vi "AlliGator Select Source Image ROI.vi"(8 "Error In":errorcluster, 11 "ROI Selection Data":T1) -> (0 "Error Out":errorcluster, 1 "Overlay Color":u32(colorbox), 2 "ROI Name":string, 3 "ROI Descriptor":T3 {"Contours"."Type" items=["No Selection", "Point", "Line", "Rectangle", "Oval", "Polygon", "Freehand Region", "Annulus", "Unused2", "Unused3", "Broken Line", "Freehand Line", "Rotated Rectangle"]}, 4 "Current ROI":i32, 5 "# ROIs":i32)   [LabVIEW 2021, in "AlliGator ROIs.lvlib"]
doc: "Selects Source Image ROI(s)."
uses:
  AlliGator ROIs.lvlib
  AlliGator ROI Selection Data.ctl
  AlliGator ROI Manager Actions.ctl
  Globals, Variables, Constants/AlliGator Variables List.ctl
  Image/Named ROI Description.ctl
  Variant/Variant to Data/Variant to I32.vi
  <userlib>/_OpenG.lib/string/string.llb/openg_string.lvlib
  Globals, Variables, Constants/AlliGator Globals, Variables & Constants.lvlib
  Image/Image.lvlib
  Variant/Variant to Data/Variant to Data.lvlib
  Arrays/Arrays.lvlib
  Utilities/Utilities.lvlib
  Time/Time.lvlib
panel:
  # "see the AlliGator License on the block diagram (Ctrl+E or Window:Show Block Diagram)"
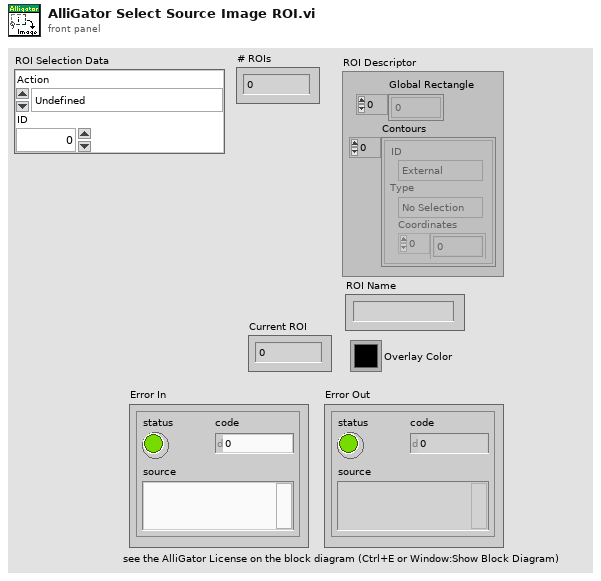
[diagram p1: front panel]
types:
  T1 = typedef "AlliGator ROIs.lvlib/AlliGator ROI Selection Data.ctl" = cluster{"Action":T2, "ID":i32}
  T2 = typedef "AlliGator ROIs.lvlib/AlliGator ROI Manager Actions.ctl" = enum16{"Undefined", "Delete Current ROI", "Delete All Unselected ROIs", "Delete Multiple ROIs", "Delete All ROIs", "Swap ROIs", "Insert ROI", "Update Current ROI Descriptor", "Rename Current ROI", "Store New ROI", "Store Multiple ROIs", "Select Next ROI", "Select Previous ROI", "Find Selected ROI", "Show All ROIs", "Update ROI Manager Window", "Merge All ROIs", "Unmerge ROI", "Set Selected ROI by ID"}
  T3 = typedef "ROI Descriptor" = cluster{"Global Rectangle":i32[], "Contours":cluster{"ID":enum32{"External", "Internal"}, "Type":u32, "Coordinates":i32[]}[]}
  T4 = typedef "AlliGator Globals, Variables & Constants.lvlib/AlliGator Variables List.ctl" = enum16{"---- GUI ----", "GUI:Initialization Status", "GUI:State Indicators Refnum", "GUI:Original AlliGator Menu Items", "GUI:Current Action Loop State", "GUI:Script in progress", "GUI:Playback", "GUI:Loop Playback", "GUI:Search ROI Used", "GUI:Search ROI", "Decay Graph Max Legend Size", "Intensity Graph Max Legend Size", "Decay Statistics Graph Max Legend Size", "Phasor Graph Max Legend Size", "Phasor Ratio Graph Max Legend Size", "Lifetime Graph Max Legend Size", "---- Files ----", "Files:Export Dataset Frames as Individual Files", "Files:Show Batch Export Help Balloons", "Files:Frames in Dataset", "Files:ptu File Frame Start Indices", "Files:Current Frame in Dataset", "Files:Current Frame Timestamp", "Files:Dataset Loaded", "Files:Dataset Metadata", "Files:Dataset Channel", "Files:Dataset Data Description", "Files:Background Dataset Metadata", "Files:Background Dataset Channel", "Files:Background Dataset Data Description", "Files:Background File Subtraction", "Files:Background File Path", "Files:Background File Pile-up Correction", "Files:Background File Pixel Well Capacity", "Files:Background File Scaling Factor", "Files:Current Dataset Load Settings", "Files:Dataset Path", "Files:ICCD-specific Information", "Files:Macrotime Gate Separation", "------ Python Plugins ------", "Python Plugins:Information", "Python Plugins:Python Session", "Python Plugins:Valid Python Session?", "---- Source Image ----", "Source Image:ROIs", "Source Image:Current ROI", "Source Image:ROI Event Refnum", "X_Source Image Display Range", "X_Source Image Palette Information", "X_Type of Displayed Image", "X_Time Gate Slider", "Source Image:Palette List", "Source Image:Scale", "Source Image:ROI Overlay Color", "Source Image:Overlay to Erase", "Source Image:Is Displayed Image Accumulated", "Source Image:White Light Image Modified", "Source Image:Mask Image Modified", "---- Image Profile Window ----", "Image Profile:Window Event Refnum", "Image Profile:IntensityType", "Image Profile:Intensity Average Type", "Image Profile:Intensity-weighted SDV", "Image Profile:Box Profile Type", "Image Profile:Window Open", "Image Profile:Plotted Fit Parameter", "------ Phasor Graph -------", "Phasor Graph:Show Line", "---- Phasor Plot ---", "Phasor Plot:Parameters Changed", "Phasor Plot:FLI Dataset Modified since last Calculation", "Phasor Harmonics Data", "Selected Phasor Harmonics", "Phasor Harmonic Manager Event Refnum", "Phasor Plot:ROIs", "Phasor Plot:Current ROI", "Phasor Plot:ROI Event Refnum", "Phasor Plot:Image Reference Points", "Phasor Plot:Computed", "Phasor Plot:Palette Information", "Phasor Plot:Palette List", "Phasor Plot:Phasor Ratio Palette Information", "Phasor Plot:Phasor Ratio Palette List", "Phasor Plot:Image Scale", "Phasor Plot:Image Overlay to Erase", "Phasor Plot:Image Elements to Update", "Phasor Plot:Current Calculation Parameters", "Phasor Plot:Current Calibration Options", "Phasor Plot:Reset Cumulated Phasor Plot", "Phasor Plot:Reference 1", "Phasor Plot:Lifetime Reference 1", "Phasor Plot:Reference 1 Frequency", "Phasor Plot:Reference 2", "Phasor Plot:Lifetime Reference 2", "Phasor Plot:Reference 2 Frequency", "---- Decay Analysis ----", "Number of Selected Decays to Fit", "LS Fit Results", "LAR Fit Results", "BS Fit Results", "Last Decay Max - Min", "Best Fit Parameters", "Best Fit Parameter Names", "Actual Size X", "Actual Size Y", "Binning X", "Binning Y", "Actual # Gates", "Dataset Number", "Gates to...", "Gates Skipped", "Gates to keep", "Gate Step", "Gate Separation", "Reversed Gates", "Pile-up Correction", "Pixel Well Capacity", "Background Subtracted", "Background Subtraction Method", "Background Definition Range", "Background File (deprecated)", "Number of Dataset Accumulated", "Array of Accumulated Dataset Paths", "Do Averaged Datasets", "Destination File Path", "Process Plot Target", "Use 1/D as Phasor Frequency", "---- Decay Fit Parameter Map -----", "Decay Fit Parameter Map:Palette Information", "Decay Fit Parameter Map:Palette List", "---- Parameter Map ----", "Parameter Map:Palette Information", "Parameter Map:Palette List", "------- Local Decay Window ---------", "Local Decay Graph Window:Event Refnum", "Local Decay Graph Window:Use normalized IRF for convolution", "----- Miscellaneous ----", "Misc:Skippable Dialog Windows Status"}
  T5 = typedef "Image.lvlib/Named ROI Description.ctl" = cluster{"ROI Descriptor":T3, "ROI Name":string, "Overlay Color":u32}
  T6 = typedef "AlliGator ROIs.lvlib/AlliGator Image ROI Event refnum.ctl" = refnum<user-event>
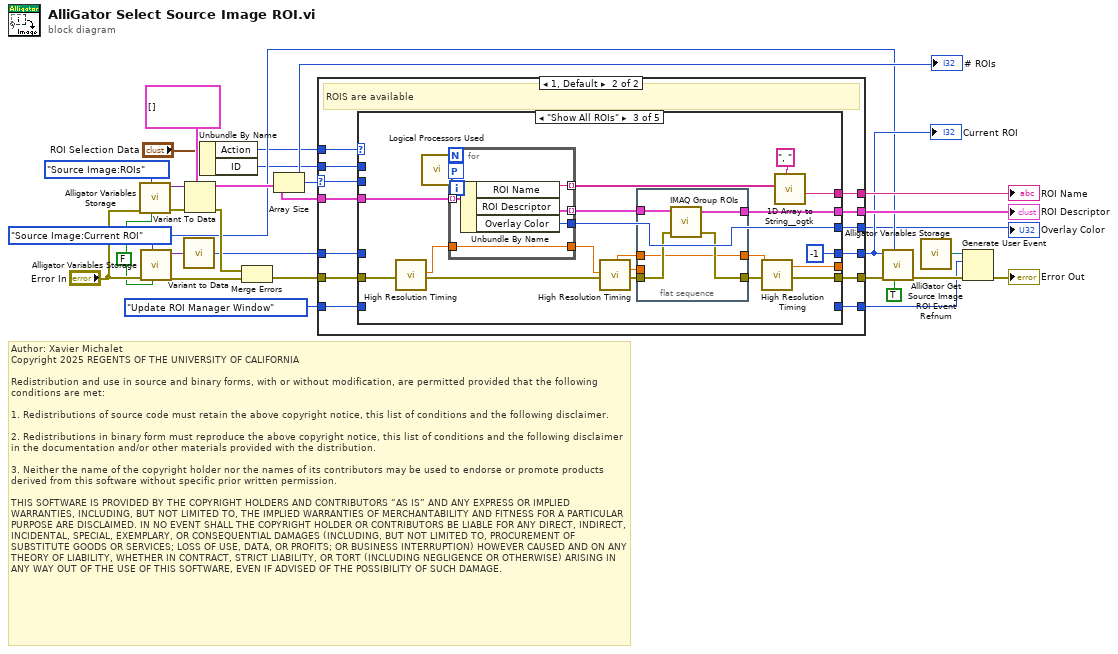
[diagram p0: block diagram]
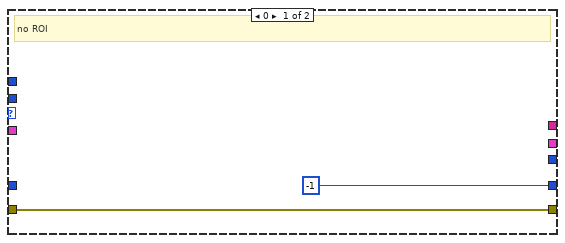
[diagram p2: hidden frame]
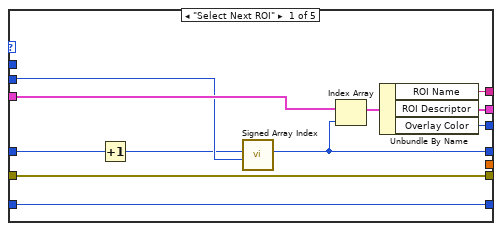
[diagram p3: hidden frame]
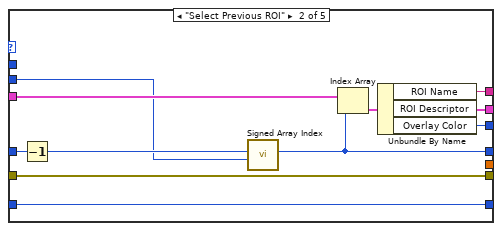
[diagram p4: hidden frame]
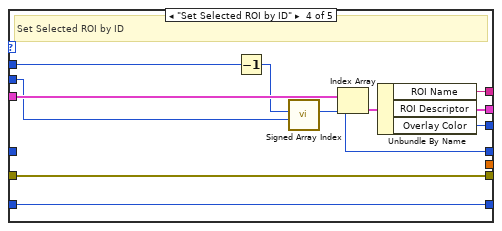
[diagram p5: hidden frame]
diagram:
  w11 = AlliGator_Variables_List."Source Image:Current ROI" ("Alligator Variable")
  w18 = FALSE ("Get(F)/Set")
  # "Author: Xavier Michalet\nCopyright 2025 REGENTS OF THE UNIVERSITY OF CALIFORNIA\n\nRedistribution and use in source and binary forms, with or without modification, are permitted provided that the following conditions are met:\n\n1. Redistributions of source code must retain the above copyright notice, this list of conditions and the following disclaimer.\n\n2. Redistributions in binary form must reproduce the above copyright notice, this list of conditions and the following disclaimer in the documentation and/or other materials provided with the distribution.\n\n3. Neither the name of the copyright holder nor the names of its contributors may be used to endorse or promote products derived from this software without specific prior written permission.\n\nTHIS SOFTWARE IS PROVIDED BY THE COPYRIGHT HOLDERS AND CONTRIBUTORS “AS IS” AND ANY EXPRESS OR IMPLIED WARRANTIES, INCLUDING, BUT NOT LIMITED TO, THE IMPLIED WARRANTIES OF MERCHANTABILITY AND FITNESS FOR A PARTICULAR PURPOSE ARE DISCLAIMED. IN NO EVENT SHALL THE COPYRIGHT HOLDER OR CONTRIBUTORS BE LIABLE FOR ANY DIRECT, INDIRECT, INCIDENTAL, SPECIAL, EXEMPLARY, OR CONSEQUENTIAL DAMAGES (INCLUDING, BUT NOT LIMITED TO, PROCUREMENT OF SUBSTITUTE GOODS OR SERVICES; LOSS OF USE, DATA, OR PROFITS; OR BUSINESS INTERRUPTION) HOWEVER CAUSED AND ON ANY THEORY OF LIABILITY, WHETHER IN CONTRACT, STRICT LIABILITY, OR TORT (INCLUDING NEGLIGENCE OR OTHERWISE) ARISING IN ANY WAY OUT OF THE USE OF THIS SOFTWARE, EVEN IF ADVISED OF THE POSSIBILITY OF SUCH DAMAGE."
  n1 = call "Alligator Variables Storage.vi"("Get(F)/Set"=w18, "AlliGator Variable"=AlliGator_Variables_List."Source Image:ROIs" ("Alligator Variable"), "Error In"="Error In") -> ("Error Out"=w23:errorcluster, "Data out"=w24:variant)  [unwired: 6 in, 1 out]
  n2 = call "Alligator Variables Storage.vi"("Get(F)/Set"=w18, "AlliGator Variable"=w11, "Error In"="Error In") -> ("Error Out"=w16:errorcluster, "Data out"=w15:variant)  [unwired: 6 in, 1 out]
  n3 = call-poly "Variant to Data.vi"("Variant"=w15) -> ("Value"=w14:i32)  [unwired: 8 in]
  n4 = Variant To Data(error in=w23, type=T5[] [] ("ROIs"), Variant=w24) -> (data=w20:T5[], error out=w21:errorcluster)
  n5 = Unbundle By Name("ROI Selection Data") -> ("Action"=w2:T2, "ID"=w1:i32)
  n6 = Merge Errors(w21, w16) -> (w17:errorcluster)
  n7 = Array Size(array=w20) -> (size(s)=w27:i32)
  "# ROIs" <- w27
  n8 = case shown="1, Default" w27 {
    selector: w27 -> [_ w32]
    tunnel: [_ w43] -> w28
    tunnel: [-1 w42] -> w13
    tunnel: w14 -> [_ w41]
    tunnel: w2 -> [_ w40]
    tunnel: w20 -> [_ w39]
    tunnel: w17 -> [w29 w38]
    tunnel: [w29 w37] -> w10
    tunnel: [_ w36] -> w26
    tunnel: [_ w35] -> w6
    tunnel: [_ w33] -> w4
    tunnel: AlliGator_ROI_Manager_Actions."Update ROI Manager Window" ("event data") -> [_ w34]
    tunnel: w1 -> [_ w31]
    frame 0 {
      # "no ROI"
    }
    frame 1, Default {
      # "ROIS are available"
      n9 = case shown="\"Show All ROIs\"" w40 {
        tunnel: w39 -> [w54 w65 w83 w106 _]
        tunnel: w41 -> [w46 w63 _ _ _]
        tunnel: [w45 w55 -1 ("Value") w98 _] -> w42
        tunnel: [w51 w61 w85 w103 _] -> w43
        tunnel: w32 -> [w47 w56 _ w99 _]
        tunnel: w38 -> [w52 w62 w84 w104 w107]
        tunnel: [w52 w62 w71 w104 w107] -> w37
        tunnel: [w50 w60 w80 w102 _] -> w36
        tunnel: [w49 w59 w78 w101 _] -> w35
        tunnel: w34 -> [w48 w58 _ w100 _]
        tunnel: [w48 w58 _ w100 _] -> w33
        tunnel: w31 -> [_ _ _ w97 _]
        tunnel: [_ _ w66 _ _] -> _
        frame "Select Next ROI" {
          n10 = Increment(x=w46) -> (x+1=w44:i32)
          n11 = call "Signed Array Index.vi"("Array Size"=w47, "Array Index in"=w44) -> ("Array Index out"=w45:i32)  [unwired: 9 in]
          n12 = Index Array(array=w54, index=w45) -> (element=w53:T5)
          n13 = Unbundle By Name(w53) -> ("ROI Name"=w50:string, "ROI Descriptor"=w51:T3, "Overlay Color"=w49:u32)
        }
        frame "Select Previous ROI" {
          n14 = Decrement(x=w63) -> (x-1=w57:i32)
          n15 = call "Signed Array Index.vi"("Array Size"=w56, "Array Index in"=w57) -> ("Array Index out"=w55:i32)  [unwired: 9 in]
          n16 = Index Array(array=w65, index=w55) -> (element=w64:T5)
          n17 = Unbundle By Name(w64) -> ("ROI Name"=w60:string, "ROI Descriptor"=w61:T3, "Overlay Color"=w59:u32)
        }
        frame "Show All ROIs" {
          n18 = call "High Resolution Timing.vi"("Error In"=w84) -> ("elapsed (relative) seconds"=w73:dbl, "Error Out"=w75:errorcluster)  [unwired: 16 in, 1 out]
          n19 = call "Logical Processors Used.vi"() -> ("# Logical Processor Used"=w76:i32)  [unwired: 6 in]
          n20 = for {
            tunnel: w83 -> [w95] mode=indexing
            tunnel: [w94] -> w82 mode=indexing
            tunnel: [w93] -> w81 mode=indexing
            tunnel: [w92] -> w78
            workers-P: w76 -> [_]
            tunnel: w73 -> [w91]
            tunnel: [w91] -> w72
            n21 = Unbundle By Name(w95) -> ("ROI Name"=w93:string, "ROI Descriptor"=w94:T3, "Overlay Color"=w92:u32)
          }
          n22 = call "High Resolution Timing.vi"("relative seconds (NaN)"=w72, "Error In"=w75) -> ("relative seconds"=w68:dbl, "elapsed (relative) seconds"=w67:dbl, "Error Out"=w74:errorcluster)  [unwired: 15 in]
          n23 = flat-sequence {
            tunnel: [w90] -> w85
            tunnel: w82 -> [w89]
            tunnel: w74 -> [w88]
            tunnel: [w87] -> w70
            tunnel: [w86] -> w69
            tunnel: w68 -> [w86]
            tunnel: w67 -> [_]
            frame #0 {
              n24 = call "IMAQ Group ROIs"("error in (no error)"=w88, "ROI Descriptors"=w89) -> ("error out"=w87:errorcluster, "ROI Descriptor out"=w90:T3)  [unwired: 2 in]
            }
          }
          n25 = call "High Resolution Timing.vi"("relative seconds (NaN)"=w69, "Error In"=w70) -> ("elapsed (relative) seconds"=w66:dbl, "Error Out"=w71:errorcluster)  [unwired: 15 in, 1 out]
          n26 = call <userlib>:"1D Array to String__ogtk.vi"("delimiter (Tab)"=", ", "Array of Strings"=w81) -> ("delimited string"=w80:string)  [unwired: 9 in]
        }
        frame "Set Selected ROI by ID" {
          # "Set Selected ROI by ID"
          n27 = Decrement(x=w97) -> (x-1=w96:i32)
          n28 = call "Signed Array Index.vi"("Array Size"=w99, "Array Index in"=w96) -> ("Array Index out"=w98:i32)  [unwired: 9 in]
          n29 = Index Array(array=w106, index=w98) -> (element=w105:T5)
          n30 = Unbundle By Name(w105) -> ("ROI Name"=w102:string, "ROI Descriptor"=w103:T3, "Overlay Color"=w101:u32)
        }
        frame Default {
        }
      }
    }
  }
  "ROI Descriptor" <- w28
  "ROI Name" <- w26
  "Overlay Color" <- w6
  "Current ROI" <- w13
  n31 = call "Alligator Variables Storage.vi"("Get(F)/Set"=TRUE, "AlliGator Variable"=w11, "Error In"=w10, "Data in"=w13) -> ("Error Out"=w8:errorcluster)  [unwired: 5 in, 2 out]
  n32 = call "AlliGator Get Source Image ROI Event Refnum.vi"() -> ("Source Image ROI Event Refnum"=w9:T6)
  n33 = Generate User Event(user event=w9, event data cluster=w4, error in=w8) -> (error out=→"Error Out":errorcluster)  [unwired: 1 in, 1 out]
